vi "Bamocar Main.vi"(8 "Error In":errorcluster) -> (0 "Error Out":errorcluster)   [LabVIEW 2018]
uses:
  TypeDefs/bamocarRegisters.ctl
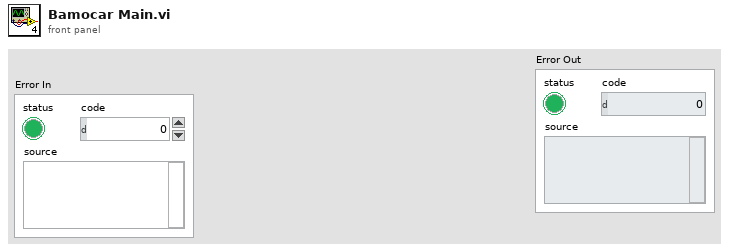
[diagram p1: front panel]
types:
  T1 = typedef "bamocarRegisters.ctl" = u16
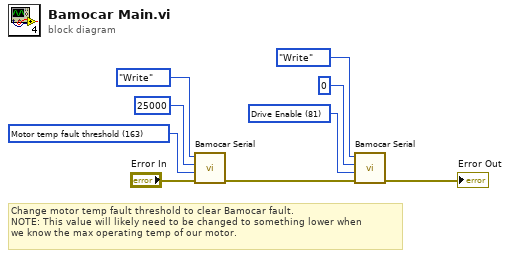
[diagram p0: block diagram]
diagram:
  w4 = T1 81 items=["Motor temp warning threshold"=162, "Motor temp fault threshold"=163, "Drive Enable"=81] ("Register")
  w7 = T1 163 items=["Motor temp warning threshold"=162, "Motor temp fault threshold"=163, "Drive Enable"=81] ("Register")
  # "Change motor temp fault threshold to clear Bamocar fault.\nNOTE: This value will likely need to be changed to something lower when \nwe know the max operating temp of our motor."
  n1 = call "Bamocar Serial.vi"("Error In"="Error In", "Register"=w7, "Value to write"=u16 25000, "Command"=enum16{"Write/Read", "Write", "Read"}."Write") -> ("Error Out"=w5:errorcluster)  [unwired: 6 in, 1 out]
  n2 = call "Bamocar Serial.vi"("Error In"=w5, "Register"=w4, "Value to write"=u16 0, "Command"=enum16{"Write/Read", "Write", "Read"}."Write") -> ("Error Out"=→"Error Out":errorcluster)  [unwired: 6 in, 1 out]
